vi "BooleanControl_Create.vi"(0 "reference in":refnum<class "BooleanControl.lvclass">, 1 "Object Attributes":T1, 2 "Control Attributes":T4, 3 "BooleanControl Attributes":T3, 5 "error in (no error)":errorcluster) -> (14 "reference out":refnum<class "BooleanControl.lvclass">, 19 "error out":errorcluster)   [LabVIEW 2014, in "BooleanControl.lvclass"]
uses:
  BooleanControl.lvclass
  Control_class/Attributes.ctl
  Text_class/Text.lvclass
  <vilib>/picture/picture.llb/imagedata.ctl
  Attributes.ctl
  Object_class/Attributes.ctl
  Object_class/Coordinates.ctl
  Control_class/Control.lvclass
  Object_class/Object.lvclass
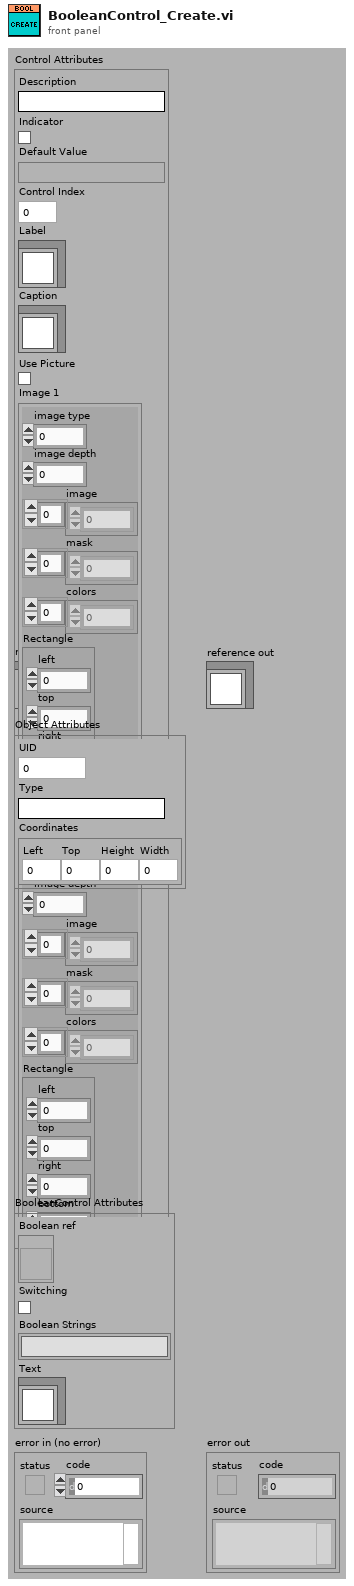
[diagram p1: front panel]
types:
  T1 = typedef "Object.lvclass/Attributes.ctl" = cluster{"UID":i32, "Type":string, "Coordinates":T2}
  T2 = typedef "Object.lvclass/Coordinates.ctl" = cluster{"Left":i32, "Top":i32, "Height":u32, "Width":u32}
  T3 = typedef "BooleanControl.lvclass/Attributes.ctl" = cluster{"Boolean ref":refnum<vi>, "Switching":bool, "Boolean Strings":string[], "Text":refnum<class "Text.lvclass">}
  T4 = typedef "Control.lvclass/Attributes.ctl" = cluster{"Description":string, "Indicator":bool, "Default Value":variant, "Control Index":i32, "Label":refnum<class "Text.lvclass">, "Caption":refnum<class "Text.lvclass">, "Use Picture":bool, "Image 1":T5, "Image 2":T5}
  T5 = typedef "imagedata.ctl" = cluster{"image type":i32, "image depth":i32, "image":u8[], "mask":u8[], "colors":u32[], "Rectangle":cluster{"left":i16, "top":i16, "right":i16, "bottom":i16}}
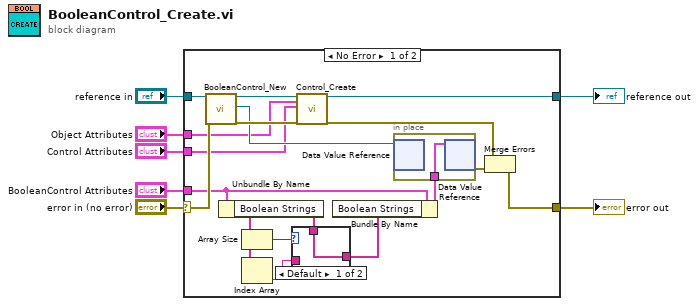
[diagram p0: block diagram]
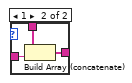
[diagram p2: hidden frame]
diagram:
  n1 = case shown="No Error" "error in (no error)" {
    selector: "error in (no error)" -> [w24 w31]
    tunnel: [w22 w31] -> w6
    tunnel: "reference in" -> [w15 w30]
    tunnel: [w19 w30] -> w4
    tunnel: "Control Attributes" -> [w17 _]
    tunnel: "BooleanControl Attributes" -> [w10 _]
    tunnel: "Object Attributes" -> [w14 _]
    frame No Error {
      n2 = call "BooleanControl_New.vi"("reference in"=w15, "error in (no error)"=w24) -> ("reference out"=w21:refnum<class "BooleanControl.lvclass">, "DVRRefOut"=w18:refnum<data-value>, "error out"=w20:errorcluster)  [unwired: 14 in, 1 out]
      n3 = Unbundle By Name(w10) -> ("Boolean Strings"=w12:string[])
      n4 = Array Size(array=w12) -> (size(s)=w13:i32)
      n5 = Index Array(array=w12) -> (element=w11:string)  [unwired: 1 in]
      n6 = case shown="Default" w13 {
        tunnel: w12 -> [w25 w28]
        tunnel: w11 -> [_ w27]
        tunnel: [w25 w26] -> w8
        frame Default {
        }
        frame 1 {
          n7 = Build Array (concatenate)(w28, w27) -> (w26:string[])
        }
      }
      n8 = call "Control_Create.vi"("reference in"=w21, "Object Attributes"=w14, "Control Attributes"=w17, "error in (no error)"=w20) -> ("reference out"=w19:refnum<class "BooleanControl.lvclass">, "error out"=w16:errorcluster)  [unwired: 14 in]
      n9 = Bundle By Name(cluster=w10, "Boolean Strings"=w8) -> (w9:T3)
      n10 = in-place {
        in-place-border: w9 -> [w29]
        n11 = in-place-dvr #1(w18) -> ()  [unwired: 2 out]
        n12 = in-place-dvr #1(w29) -> (w23:errorcluster)  [unwired: 1 out]
      }
      n13 = Merge Errors(w16, w23) -> (w22:errorcluster)
    }
    frame Error {
    }
  }
  "error out" <- w6
  "reference out" <- w4
